vi "timing.vi"(8 "error in (no error)":errorcluster, 10 "input complex waveform":cluster{"t0":dbl, "dt":dbl, "Y":cdb[]}={"t0"=0.0, "dt"=1.0, "Y"=[]} {"Y" format="%.3f"; "dt" format="%^.2e"; "t0" format="%.4f"}, 11 "Modulation Parameters In":T1={"RX Parameters"={"RX Oversample Factor"=4, "RX Sample Rate"=4000000.0, "Synchronization Options"={"Synchronization Method"=enum."Fixed Offset", "Symbol Timing Recovery Method "=enum."MT Allign To Ideal Symbols", "Fixed Offset"=0, "Frame Detection Method"=enum."", "Correct Frequency Offset"=FALSE}, "Channel Estimation/Equalization Parameters"={"Equalization Method"=enum."", "Channel Estimate Length"=0.0, "Equalizer Length"=0.0, "Equalizer Delay"=0.0}}, "TX/RX Shared Parameters"={"Modulation Type"=enum."OOK", "Packet Length"=128, "# of Iterations"=0.0, "Pulse Shaping Parameters"={"Pulse Shaping Filter"=enum."none", "Filter Length (symbols)"=32, "Filter Parameter"=0.8, "modulation type"=enum."FSK"}, "Header/Tail Control Information"={"Training Sequence Type"=enum."", "Zero Pad Length"=0.0}}}) -> (0 "error out":errorcluster, 1 "alignment offset (samples)":i32, 2 "output complex waveform":cluster{"t0":dbl, "dt":dbl, "Y":cdb[]}, 3 "Modulation Parameters Out":T1={"RX Parameters"={"RX Oversample Factor"=4, "RX Sample Rate"=4000000.0, "Synchronization Options"={"Synchronization Method"=enum."Fixed Offset", "Symbol Timing Recovery Method "=enum."MT Allign To Ideal Symbols", "Fixed Offset"=0, "Frame Detection Method"=enum."", "Correct Frequency Offset"=FALSE}, "Channel Estimation/Equalization Parameters"={"Equalization Method"=enum."", "Channel Estimate Length"=0.0, "Equalizer Length"=0.0, "Equalizer Delay"=0.0}}, "TX/RX Shared Parameters"={"Modulation Type"=enum."OOK", "Packet Length"=128, "# of Iterations"=0.0, "Pulse Shaping Parameters"={"Pulse Shaping Filter"=enum."none", "Filter Length (symbols)"=32, "Filter Parameter"=0.8, "modulation type"=enum."FSK"}, "Header/Tail Control Information"={"Training Sequence Type"=enum."", "Zero Pad Length"=0.0}}})   [LabVIEW 2012]
uses:
  <vilib>/Analysis/2dsp.llb/Decimate (single shot, CDB).vi
  <vilib>/addons/Modulation/Digital/General/MT Align to Ideal Symbols (Generic).vi
  <vilib>/Analysis/NI_AALPro.lvlib
  <vilib>/addons/Modulation/niDMT.lvlib
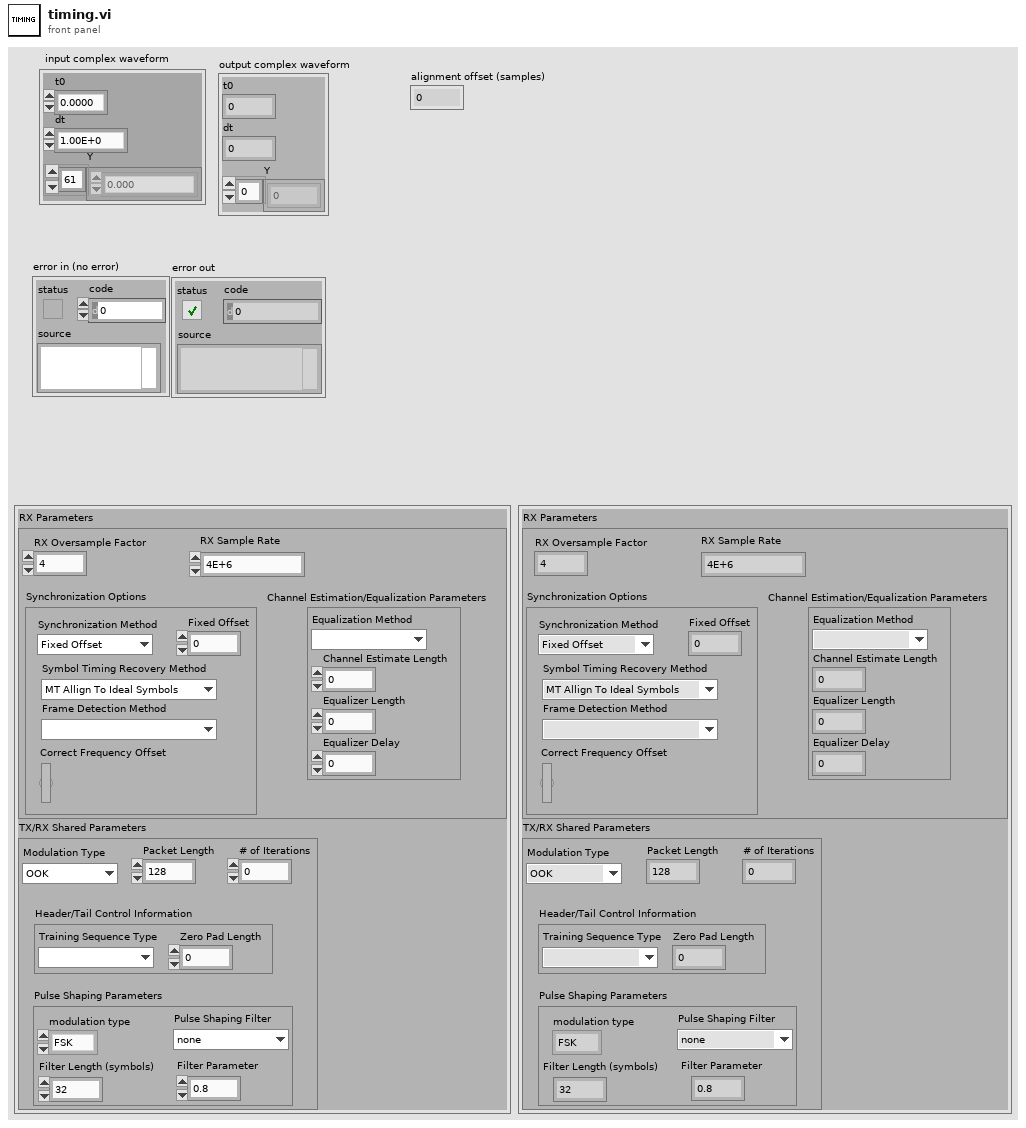
[diagram p1: front panel]
types:
  T1 = cluster{"RX Parameters":cluster{"RX Oversample Factor":i32, "RX Sample Rate":dbl, "Synchronization Options":cluster{"Synchronization Method":enum16{"Fixed Offset", "Timing Estimation", "Joint Timing and Channel Estimation"}, "Symbol Timing Recovery Method ":enum16{"MT Allign To Ideal Symbols", "Maximum Energy", "Early-Late Gate", "Gardner", "Fixed Offset"}, "Fixed Offset":i32, "Frame Detection Method":enum16{""}, "Correct Frequency Offset":bool}, "Channel Estimation/Equalization Parameters":cluster{"Equalization Method":enum16{""}, "Channel Estimate Length":dbl, "Equalizer Length":dbl, "Equalizer Delay":dbl}}, "TX/RX Shared Parameters":cluster{"Modulation Type":enum16{"OOK", "FSK"}, "Packet Length":i32, "# of Iterations":dbl, "Pulse Shaping Parameters":cluster{"Pulse Shaping Filter":enum16{"none", "Raised Cosine", "Root Raised Cos", "Gaussian"}, "Filter Length (symbols)":i32, "Filter Parameter":dbl, "modulation type":enum16{"FSK", "PSK", "QAM", "MSK", "PAM", "ASK", "CPM"}}, "Header/Tail Control Information":cluster{"Training Sequence Type":enum16{""}, "Zero Pad Length":dbl}}}
  T2 = enum16{"MT Allign To Ideal Symbols", "Maximum Energy", "Early-Late Gate", "Gardner", "Fixed Offset"}
  T3 = cluster{"Pulse Shaping Filter":enum16{"none", "Raised Cosine", "Root Raised Cos", "Gaussian"}, "Filter Length (symbols)":i32, "Filter Parameter":dbl, "modulation type":enum16{"FSK", "PSK", "QAM", "MSK", "PAM", "ASK", "CPM"}}
  T4 = enum16{"FSK", "PSK", "QAM", "MSK", "PAM", "ASK", "CPM"}
  T5 = enum16{"none", "Raised Cosine", "Root Raised Cos", "Gaussian"}
  T6 = typedef "niAMT.lvlib/Complex Data Waveform.ctl" = cluster{"t0":dbl, "dt":dbl, "Y":cdb[]}
  T7 = cluster{"RX Parameters":cluster{"RX Oversample Factor":i32, "RX Sample Rate":dbl, "Synchronization Options":cluster{"Synchronization Method":enum16{"Fixed Offset", "Timing Estimation", "Joint Timing and Channel Estimation"}, "Symbol Timing Recovery Method ":enum16{"MT Allign To Ideal Symbols", "Maximum Energy", "Early-Late Gate", "Gardner", "Fixed Offset"}, "Fixed Offset":dbl, "Frame Detection Method":enum16{""}, "Correct Frequency Offset":bool}, "Channel Estimation/Equalization Parameters":cluster{"Equalization Method":enum16{""}, "Channel Estimate Length":dbl, "Equalizer Length":dbl, "Equalizer Delay":dbl}}, "TX/RX Shared Parameters":cluster{"Modulation Type":enum16{"OOK", "FSK"}, "Packet Length":i32, "# of Iterations":dbl, "Pulse Shaping Parameters":cluster{"Pulse Shaping Filter":enum16{"none", "Raised Cosine", "Root Raised Cos", "Gaussian"}, "Filter Length (symbols)":i32, "Filter Parameter":dbl, "modulation type":enum16{"FSK", "PSK", "QAM", "MSK", "PAM", "ASK", "CPM"}}, "Header/Tail Control Information":cluster{"Training Sequence Type":enum16{""}, "Zero Pad Length":dbl}}}
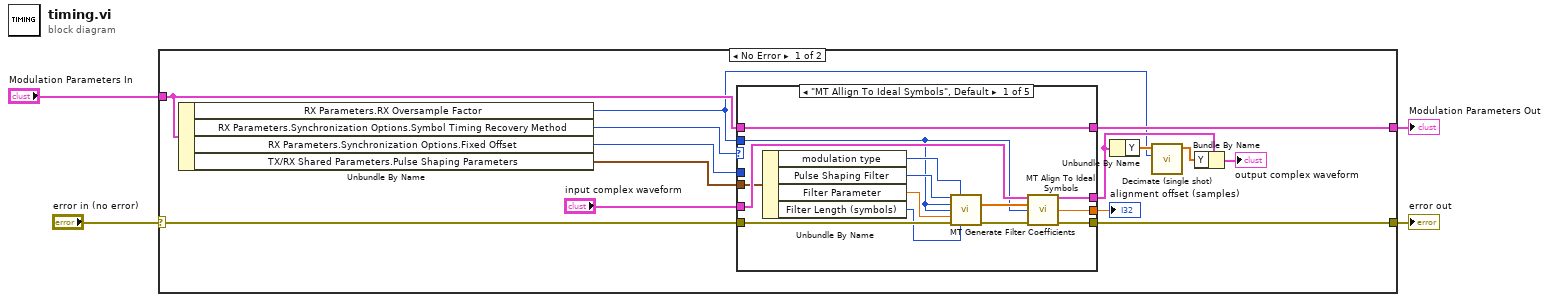
[diagram p0: block diagram]
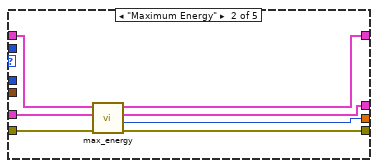
[diagram p2: hidden frame]
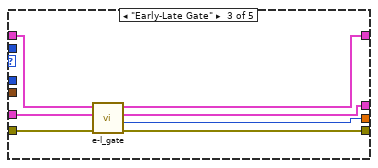
[diagram p3: hidden frame]
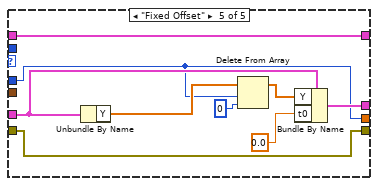
[diagram p5: hidden frame]
diagram:
  n1 = case shown="No Error" "error in (no error)" {
    selector: "error in (no error)" -> [w16 w61]
    tunnel: "Modulation Parameters In" -> [w11 w60]
    tunnel: [w15 w61] -> w3
    tunnel: [w10 w60] -> w1
    frame No Error {
      n2 = Unbundle By Name(w11) -> ("RX Parameters.RX Oversample Factor"=w5:i32, "RX Parameters.Synchronization Options.Symbol Timing Recovery Method"=w18:T2, "RX Parameters.Synchronization Options.Fixed Offset"=w7:i32, "TX/RX Shared Parameters.Pulse Shaping Parameters"=w6:T3)
      n3 = case shown="\"MT Allign To Ideal Symbols\", Default" w18 {
        tunnel: "input complex waveform" -> [w28 w36 w44 w49 w57]
        tunnel: w11 -> [w20 w35 w45 w50 w54]
        tunnel: w16 -> [w26 w39 w42 w48 w51]
        tunnel: [w31 w38 w41 w48 w51] -> w15
        tunnel: [w32 w37 w43 w49 w55] -> w12
        tunnel: [w20 w34 w46 w50 w54] -> w10
        tunnel: [w30 w33 w40 w47 w52] -> w8
        tunnel: w7 -> [_ _ _ w47 w52]
        tunnel: w6 -> [w25 _ _ _ _]
        tunnel: w5 -> [w19 _ _ _ _]
        frame "MT Allign To Ideal Symbols", Default {
          n4 = Unbundle By Name(w25) -> ("modulation type"=w24:T4, "Pulse Shaping Filter"=w23:T5, "Filter Parameter"=w22:dbl, "Filter Length (symbols)"=w21:i32)
          n5 = call <vilib>:"MT Generate Filter Coefficients.vi"("pulse shaping filter (none)"=w23, "modulation type"=w24, "pulse shaping samples per symbol (16)"=w19, "matched samples per symbol (16)"=w19, "filter parameter"=w22, "error in (no error)"=w26, "filter length (symbols)"=w21) -> ("matched filter coefficients"=w29:dbl[], "error out"=w27:errorcluster)  [unwired: 6 in, 1 out]
          n6 = call-poly <vilib>:"MT Align To Ideal Symbols.vi"("input complex waveform"=w28, "matched filter coefficients"=w29, "samples per symbol (16)"=w19, "error in (no error)"=w27) -> ("output complex waveform"=w32:T6, "waveform alignment offset (samples)"=w30:dbl, "error out"=w31:errorcluster)  [unwired: 9 in]
        }
        frame "Maximum Energy" {
          n7 = call "max_energy.vi"("error in (no error)"=w39, "input complex waveform"=w36, "Modulation Parameters In"=w35) -> ("error out"=w38:errorcluster, "alignment offset (samples)"=w33:i32, "aligned complex waveform"=w37:cluster{"t0":dbl, "dt":dbl, "Y":cdb[]}, "Modulation Parameters Out"=w34:T7)  [unwired: 5 in]
        }
        frame "Early-Late Gate" {
          n8 = call "e-l_gate.vi"("error in (no error)"=w42, "input complex waveform"=w44, "Modulation Parameters In"=w45) -> ("error out"=w41:errorcluster, "alignment offset (samples)"=w40:i32, "aligned complex waveform"=w43:cluster{"t0":dbl, "dt":dbl, "Y":cdb[]}, "Modulation Parameters Out"=w46:T7)  [unwired: 5 in]
        }
        frame "Gardner" {
          # "To be implemented"
        }
        frame "Fixed Offset" {
          n9 = Unbundle By Name(w57) -> ("Y"=w59:cdb[])
          n10 = Delete From Array(array=w59, length=w52, index=0) -> (array with subset deleted=w56:cdb[])  [unwired: 1 out]
          n11 = Bundle By Name(cluster=w57, "Y"=w56, "t0"=0.0) -> (w55:cluster{"t0":dbl, "dt":dbl, "Y":cdb[]})
        }
      }
      "alignment offset (samples)" <- w8
      n12 = Unbundle By Name(w12) -> ("Y"=w14:cdb[])
      n13 = call-poly <vilib>:"Decimate (single shot).vi"("decimating factor"=w5, "X"=w14) -> ("Decimated Array"=w13:cdb[])  [unwired: 8 in, 1 out]
      n14 = Bundle By Name(cluster=w12, "Y"=w13) -> (→"output complex waveform":T6)
    }
    frame Error {
    }
  }
  "error out" <- w3
  "Modulation Parameters Out" <- w1
